vi "ActDriveStraight.vi"(9 "FirstTime":bool, 10 "MaxSpeed (ft/s)":dbl, 11 "Dist (ft)":dbl) -> (1 "XSpeedDemand":dbl, 3 "Done":bool)   [LabVIEW 2023]
doc: "Robot will drive forward straight a set distance utilizing position control \n\nInputs:\n-- MaxSpeed -- Double -- in ft/s, the MaxSpeed the robot can go -- \n-- Dist (ft) -- Double -- Distance in feet you want the robot to go -- \n-- FirstTime -- Boolean -- Input true the first time this function is called, sets the target position -- \n\nOutputs:\n-- Done -- Bool -- has the robot reached its target distance\n-- LeftSpeedDemand -- Double -- Speed Demand for left drive train inorder to reach target -- \n-- RightSpeedDemand -- Double -- Speed Demand for left drive train inorder to reach target --"
uses:
  <vilib>/Rock Robotics/WPI/ThirdParty/JAS_Junk/TrajLib/Trajectory_Library.lvlib
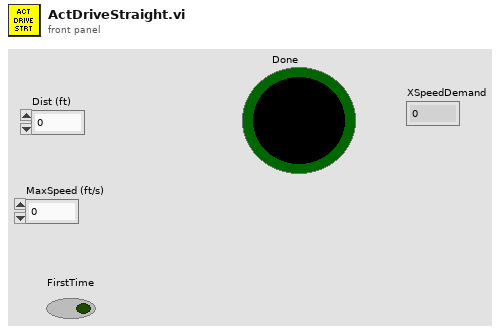
[diagram p1: front panel]
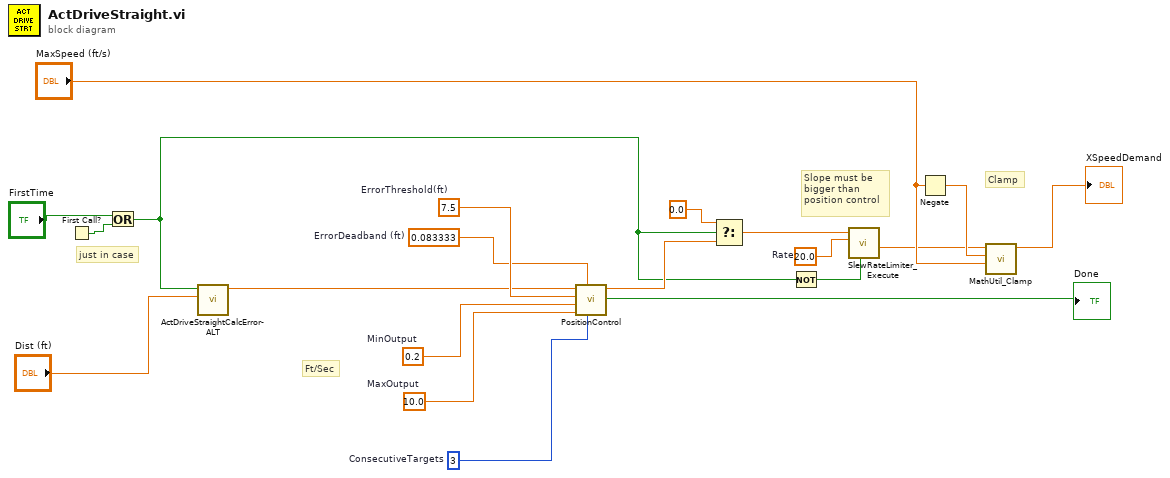
[diagram p0: block diagram]
diagram:
  w9 = 20.0  # Rate
  w13 = 10.0  # MaxOutput
  w14 = 0.2  # MinOutput
  w17 = 3  # ConsecutiveTargets
  w18 = 0.083333  # ErrorDeadband (ft)
  w19 = 7.5  # ErrorThreshold(ft)
  # "just in case"
  # "Slope must be\nbigger than\nposition control"
  # "Ft/Sec"
  # "Clamp"
  n1 = First Call?() -> (First Call?: T/F=w2:bool)
  n2 = Or(x="FirstTime", y=w2) -> (x .or. y?=w1:bool)
  n3 = call "ActDriveStraightCalcError-ALT.vi"("Dist (ft)"="Dist (ft)", "FirstTime"=w1) -> ("Dist Error (Ft)"=w11:dbl)  [unwired: 9 in]
  n4 = call "PositionControl.vi"("ConsecutiveTargets"=w17, "ErrorDeadband"=w18, "MaxOutput"=w13, "MinOutput"=w14, "ErrorThreshold"=w19, "Error"=w11) -> ("OnTarget"=→"Done":bool, "OutputValue"=w8:dbl)  [unwired: 3 in, 1 out]
  n5 = Select(t=0.0, s=w1, f=w8) -> (s? t:f=w6:dbl)
  n6 = Not(x=w1) -> (.not. x?=w5:bool)
  n7 = call <vilib>:"SlewRateLimiter_Execute.vi"("Enable"=w5, "PositiveRate"=w9, "Input"=w6) -> ("Output"=w4:dbl)  [unwired: 7 in, 1 out]
  n8 = Negate(x="MaxSpeed (ft/s)") -> (-x=w16:dbl)
  n9 = call <vilib>:"MathUtil_Clamp.vi"("High Limit"="MaxSpeed (ft/s)", "Low Limit"=w16, "Value"=w4) -> ("Result"=→"XSpeedDemand":dbl)  [unwired: 8 in]
